vi "TSM SSC DAQmx Write Mic Sensitivity Per-Site Per-Pin.vi"(0 "DAQ TSM in":T1, 1 "Idle Channel Value (0)":dbl, 5 "Per-Site Per-Pin Mic Sensitivity in":dbl[][](array[numeric]), 11 "error in":errorcluster) -> (4 "DAQ TSM Out":T1, 15 "error out":errorcluster)   [LabVIEW 2020]
doc: "Writes one or more Sensitivity to a task that contains one or more analog output channels. The Sensitivity(mV/Pa) data should be in the same order as SSC."
uses:
  Pin Map/TSM DAQmx Multi-Task.ctl
  <vilib>/NI_TestStand_SemiconductorModule/NI_TestStand_Semiconductor_Module.lvlibp/PinMap/PinQueryContext/MultiplePinMultipleSessionQueryContext/MultiplePinMultipleSessionQueryContext.lvclass
  Pin Map/SSC DAQmx.ctl
  523e543d-0678-41ee-875f-de7ba3d8a92e.vi
  <resource>/objmgr/daqmx.rc
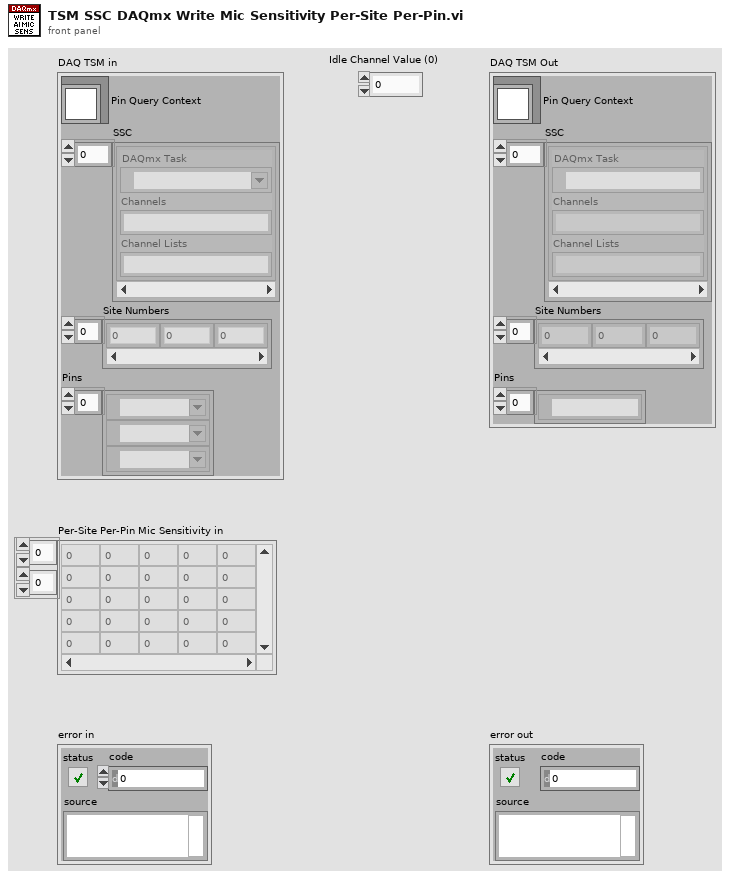
[diagram p1: front panel]
types:
  T1 = typedef "TSM DAQmx Multi-Task.ctl" = cluster{"Pin Query Context":refnum<class "MultiplePinMultipleSessionQueryContext.lvclass">, "SSC":T2[], "Site Numbers":i32[], "Pins":tag[]}
  T2 = typedef "SSC DAQmx.ctl" = cluster{"DAQmx Task ":refnum<k21>, "Channels":string, "Channel Lists":string}
  T3 = typedef "Digital 2D Location.ctl" = cluster{"Row":i32, "Col":i32}
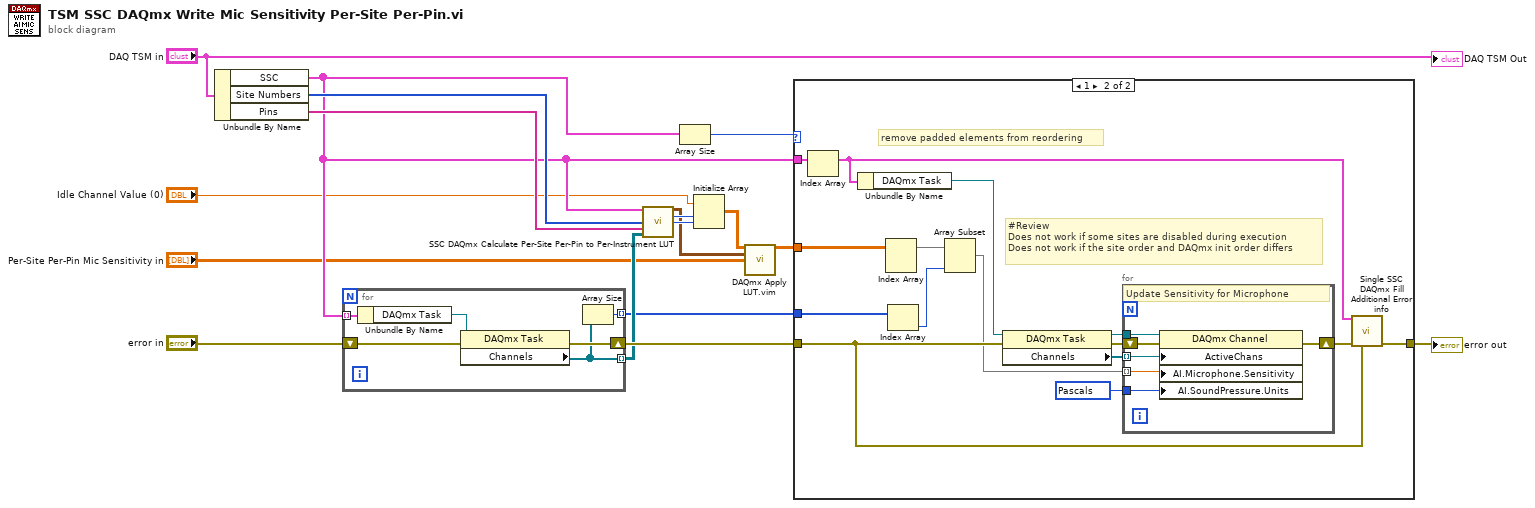
[diagram p0: block diagram]
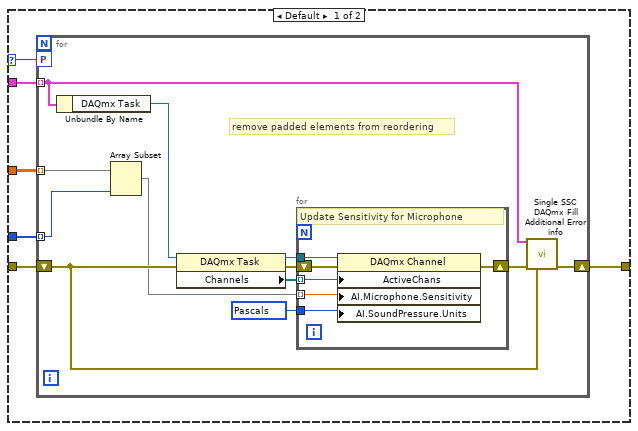
[diagram p2: hidden frame]
diagram:
  n1 = Unbundle By Name("DAQ TSM in") -> ("SSC"=w5:T2[], "Site Numbers"=w14:i32[], "Pins"=w13:tag[])
  n2 = for {
    shift-right: [w22] -> w6
    shift-left: "error in" -> [w23]
    tunnel: w5 -> [w21] mode=indexing
    tunnel: [w19] -> w4 mode=indexing
    tunnel: [w18] -> w3 mode=indexing
    n3 = Unbundle By Name(w21) -> ("DAQmx Task"=w20:refnum<k21>)
    n4 = property class="DAQmx Task"(reference=w20, error in=w23) -> (error out=w22:errorcluster, "Channels"=w19:refnum<k21>[])  [unwired: 1 out]
    n5 = Array Size(array=w19) -> (size(s)=w18:i32)
  }
  n6 = call "SSC DAQmx Calculate Per-Site Per-Pin to Per-Instrument LUT.vi"("DAQmx SSC in"=w5, "Sites"=w14, "Pins"=w13, "AO Channels"=w4) -> ("Per-Site Per-Pin to Per-Task LUT"=w10:T3[][], "Task Count"=w12:i32, "Max Channels in a Task"=w11:i32)  [unwired: 9 in]
  n7 = Array Size(array=w5) -> (size(s)=w7:i32)
  n8 = Initialize Array("Idle Channel Value (0)", w12, w11) -> (w9:dbl[][])
  n9 = call "DAQmx Apply LUT.vim"("Initialized Array"=w9, "LUT"=w10, "Results to Apply LUT to"="Per-Site Per-Pin Mic Sensitivity in") -> ("Array Out"=w8:dbl[][])  [unwired: 12 in]
  n10 = case shown="1" w7 {
    selector: w7 -> [w27 _]
    tunnel: [w29 w62] -> w15
    tunnel: w6 -> [w28 w51]
    tunnel: w5 -> [w26 w61]
    tunnel: w8 -> [w25 w60]
    tunnel: w3 -> [w24 w59]
    frame Default {
      n11 = for {
        tunnel: w26 -> [w40] mode=indexing
        workers-P: w27 -> [_]
        shift-right: [w41] -> w29
        shift-left: w28 -> [w36]
        tunnel: w25 -> [w39] mode=indexing
        tunnel: w24 -> [w38] mode=indexing
        w30 = 10081 items=["Pascals"=10081, "From Custom Scale"=10065] ("AI.SoundPressure.Units")
        # "remove padded elements from reordering"
        n12 = Unbundle By Name(w40) -> ("DAQmx Task"=w37:refnum<k21>)
        n13 = Array Subset(array=w39, length=w38) -> (w32:dbl[])  [unwired: 1 in]
        n14 = property class="DAQmx Task"(reference=w37, error in=w36) -> (reference out=w34:refnum<k21>, error out=w35:errorcluster, "Channels"=w33:refnum<k21>[])
        n15 = for {
          tunnel: w34 -> [w46]
          tunnel: w33 -> [w45] mode=indexing
          tunnel: w32 -> [w44] mode=indexing
          shift-right: [w43] -> w31
          shift-left: w35 -> [w47]
          tunnel: w30 -> [w42]
          # "Update Sensitivity for Microphone"
          n16 = property class="DAQmx Channel"(reference=w46, error in=w47, "ActiveChans"=w45, "AI.Microphone.Sensitivity"=w44, "AI.SoundPressure.Units"=w42) -> (error out=w43:errorcluster)  [unwired: 1 out]
        }
        n17 = call "Single SSC DAQmx Fill Additional Error info.vi"("DAQmx SSC in"=w40, "error in"=w31, "previous error in"=w36) -> ("error out"=w41:errorcluster)  [unwired: 12 in]
      }
    }
    frame 1 {
      w48 = 10081 items=["Pascals"=10081, "From Custom Scale"=10065] ("AI.SoundPressure.Units")
      # "#Review\nDoes not work if some sites are disabled during execution\nDoes not work if the site order and DAQmx init order differs"
      # "remove padded elements from reordering"
      n18 = Index Array(array=w61) -> (element=w58:T2)  [unwired: 1 in]
      n19 = Unbundle By Name(w58) -> ("DAQmx Task"=w49:refnum<k21>)
      n20 = Index Array(array=w60) -> (element=w56:dbl[])  [unwired: 2 in]
      n21 = Index Array(array=w59) -> (element=w57:i32)  [unwired: 1 in]
      n22 = Array Subset(array=w56, length=w57) -> (w50:dbl[])  [unwired: 1 in]
      n23 = property class="DAQmx Task"(reference=w49, error in=w51) -> (reference out=w54:refnum<k21>, error out=w55:errorcluster, "Channels"=w53:refnum<k21>[])
      n24 = for {
        tunnel: w54 -> [w67]
        tunnel: w53 -> [w66] mode=indexing
        tunnel: w50 -> [w65] mode=indexing
        shift-right: [w64] -> w52
        shift-left: w55 -> [w68]
        tunnel: w48 -> [w63]
        # "Update Sensitivity for Microphone"
        n25 = property class="DAQmx Channel"(reference=w67, error in=w68, "ActiveChans"=w66, "AI.Microphone.Sensitivity"=w65, "AI.SoundPressure.Units"=w63) -> (error out=w64:errorcluster)  [unwired: 1 out]
      }
      n26 = call "Single SSC DAQmx Fill Additional Error info.vi"("DAQmx SSC in"=w58, "error in"=w52, "previous error in"=w51) -> ("error out"=w62:errorcluster)  [unwired: 12 in]
    }
  }
  "error out" <- w15
  "DAQ TSM Out" <- "DAQ TSM in"
